vi "例4-2.vi"() -> ()   [LabVIEW 2019]
panel:
  out "MIN":dbl format="%_5g"
  out "MAX":dbl format="%_6g"
  in  "N":dbl=30.0
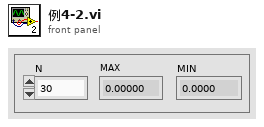
[diagram p1: front panel]
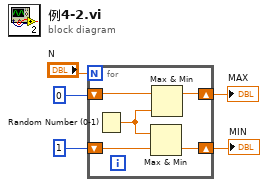
[diagram p0: block diagram]
diagram:
  n1 = for {
    N: "N" -> [_]
    shift-right: [w7] -> w1
    shift-left: 0 -> [w10]
    shift-right: [w6] -> w2
    shift-left: 1 -> [w8]
    n2 = Random Number (0-1)() -> (number: 0 to 1=w9:dbl)
    n3 = Max & Min(x=w9, y=w8) -> (min(x,y)=w6:dbl)  [unwired: 1 out]
    n4 = Max & Min(x=w10, y=w9) -> (max(x,y)=w7:dbl)  [unwired: 1 out]
  }
  "MAX" <- w1
  "MIN" <- w2
